vi "Launch Service.vi"(8 "error in (no error)":errorcluster, 10 "Topic":string, 11 "Pub Sub Message Channel":refnum<class "Pub Sub Message Channel.lvclass">) -> (0 "error out":errorcluster, 2 "Enqueuer":refnum<class "Message Enqueuer.lvclass">, 3 "Pub Sub Message Channel Out":refnum<class "Pub Sub Message Channel.lvclass">)   [LabVIEW 2020, in "Actor Pub Sub Channels.lvlib" / "Pub Sub Message Channel.lvclass"]
uses:
  Pub Sub Message Channel.lvclass
  Service Wrapper.vi
  Pub Sub Message Channel.lvclass/Pub Sub Message Channel.ctl
  <vilib>/ActorFramework/Message Enqueuer/Message Enqueuer.lvclass
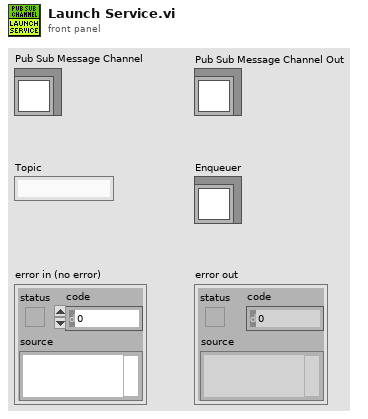
[diagram p1: front panel]
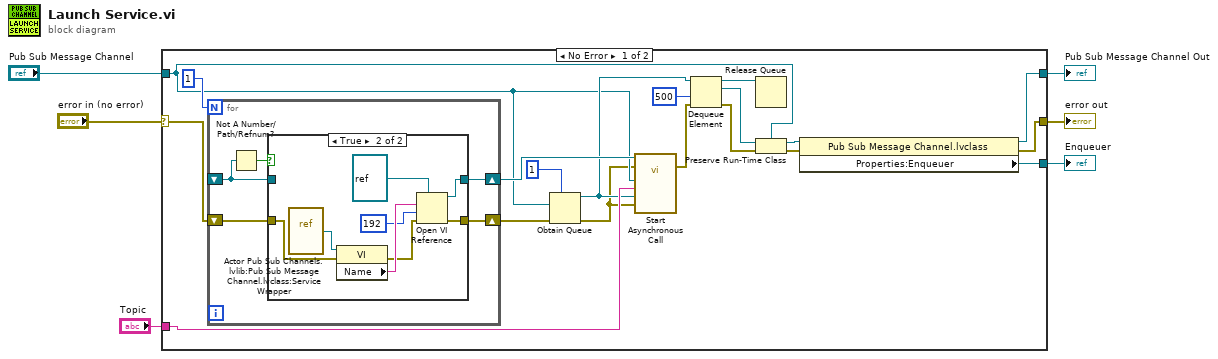
[diagram p0: block diagram]
diagram:
  n1 = case shown="No Error" "error in (no error)" {
    selector: "error in (no error)" -> [w13 w42]
    tunnel: [w10 w42] -> w5
    tunnel: "Pub Sub Message Channel" -> [w15 w41]
    tunnel: "Topic" -> [w23 _]
    tunnel: [w8 w41] -> w2
    tunnel: [w7 _] -> w1
    frame No Error {
      n2 = for {
        N: 1 -> [_]
        shift-right: [w29] -> w12
        shift-left: w13 -> [w28]
        shift-right: [w30] -> w25
        shift-left: _ -> [w26]
        n3 = Not A Number/Path/Refnum?(number/path/refnum=w26) -> (NaN/Path/Refnum?=w27:bool)
        n4 = case shown="True" w27 {
          tunnel: [w32 w38] -> w30
          tunnel: [w31 w37] -> w29
          tunnel: w28 -> [w31 w35]
          tunnel: w26 -> [w32 _]
          frame False {
          }
          frame True {
            n5 = vi-ref "Actor Pub Sub Channels.lvlib:Pub Sub Message Channel.lvclass:Service Wrapper.vi"() -> (w40:refnum<vi>)
            n6 = property class="VI"(reference=w40, error in=w35) -> (error out=w36:errorcluster, "Name"=w39:string)  [unwired: 1 out]
            n7 = Open VI Reference(type specifier VI Refnum (for type only)=refnum<vi> refnum, vi path=w39, options=192, error in (no error)=w36) -> (vi reference=w38:refnum<vi>, error out=w37:errorcluster)  [unwired: 2 in]
          }
        }
      }
      n8 = Obtain Queue(max queue size (-1, unlimited)=1, element data type=w15, error in (no error)=w12) -> (queue out=w20:refnum<queue>, error out=w11:errorcluster)  [unwired: 2 in, 1 out]
      n9 = call-by-ref "Start Asynchronous Call"(reference=w25, error in=w11, 8:"error in (no error)"=w11, "queue out"=w20, "Topic"=w23, "Pub Sub Message Channel in"=w15) -> (error out=w21:errorcluster)  [unwired: 6 in, 3 out]
      n10 = Dequeue Element(queue=w20, timeout in ms (-1)=500, error in (no error)=w21) -> (queue out=w14:refnum<queue>, element=w16:refnum<class "Pub Sub Message Channel.lvclass">, error out=w18:errorcluster)  [unwired: 1 out]
      n11 = Release Queue(queue=w14) -> ()  [unwired: 2 in, 3 out]
      n12 = Preserve Run-Time Class(object in=w16, error in=w18, 2:w15) -> (object out=w9:refnum<class "Pub Sub Message Channel.lvclass">, error out=w17:errorcluster)
      n13 = property class="Pub Sub Message Channel.lvclass"(reference=w9, error in=w17) -> (reference out=w8:refnum<class "Pub Sub Message Channel.lvclass">, error out=w10:errorcluster, "Properties:Enqueuer"=w7:refnum<class "Message Enqueuer.lvclass">)
    }
    frame Error {
    }
  }
  "error out" <- w5
  "Pub Sub Message Channel Out" <- w2
  "Enqueuer" <- w1
